vi "Do.vi"(8 "error in (no error)":errorcluster, 10 "Actor in":refnum<class "Actor.lvclass">, 11 "Launch Nested Panel Message Msg in":refnum<class "Launch Nested Panel Message Msg.lvclass">) -> (0 "error out":errorcluster, 2 "Actor out":refnum<class "Actor.lvclass">)   [LabVIEW 2023, in "Panel Actor.lvlib" / "Launch Nested Panel Message Msg.lvclass"]
doc: "(<B>Filename</B>: Actor Framework.lvlib:Message.lvclass:Do.vi)\n\nDefines what a message does when it is received by an actor. Generally, a message instructs an actor to invoke one of its methods. By default, this method does nothing. A child class must override it to define behavior. Create a child class by using the Actor Framework Message Maker dialog box."
uses:
  Launch Nested Panel Message Msg.lvclass
  builds/Framework/Actor Framework.lvlibp/1abvi3w/vi.lib/ActorFramework/Actor/Actor.lvclass
  Library/Panel Actor.lvclass
  C:/Users/Public/Documents/Development/builds/Framework/Actor Framework.lvlibp/1abvi3w/vi.lib/ActorFramework/Actor/Actor.lvclass
  Launch Nested Panel Message Msg.lvclass/Launch Nested Panel Message Msg.ctl
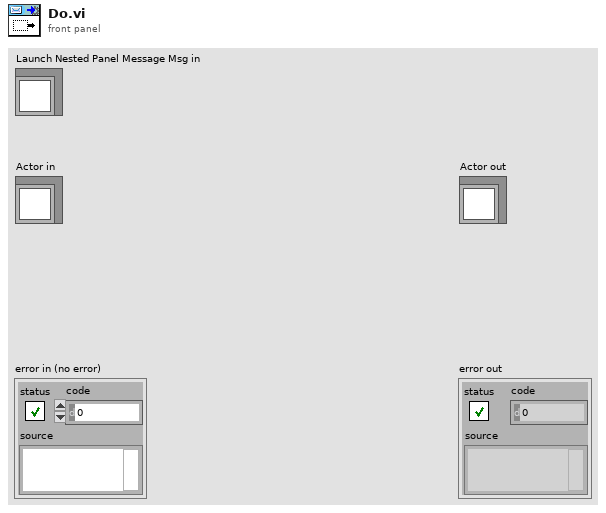
[diagram p1: front panel]
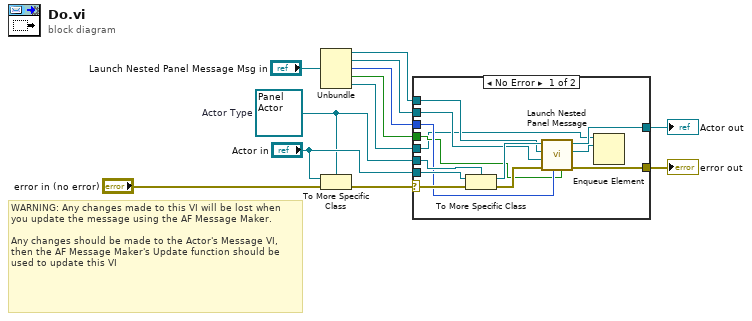
[diagram p0: block diagram]
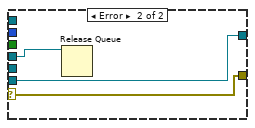
[diagram p2: hidden frame]
diagram:
  w7 = refnum<class "Panel Actor.lvclass"> refnum  # Actor Type
  # "WARNING: Any changes made to this VI will be lost when you update the message using the AF Message Maker.\n\nAny changes should be made to the Actor's Message VI, then the AF Message Maker's Update function should be used to update this VI"
  n1 = Unbundle("Launch Nested Panel Message Msg in") -> (w6:refnum<class "Panel Actor.lvclass">, w5:refnum<class "Panel.lvclass">, w4:i32, w3:bool, w1:refnum<queue>)
  n2 = To More Specific Class(target class=w7, reference="Actor in", error in="error in (no error)") -> (error out=w11:errorcluster)  [unwired: 1 out]
  n3 = case shown="No Error" w11 {
    selector: w11 -> [w25 w28]
    tunnel: [w20 w28] -> w10
    tunnel: [w19 w27] -> w9
    tunnel: "Actor in" -> [w24 w27]
    tunnel: w7 -> [w23 _]
    tunnel: w6 -> [w18 _]
    tunnel: w5 -> [w17 _]
    tunnel: w4 -> [w16 _]
    tunnel: w3 -> [w15 _]
    tunnel: w1 -> [w14 w26]
    frame No Error {
      n4 = To More Specific Class ("Actor Cast")(target class=w23, reference=w24, error in=w25) -> (specific class reference=w22:refnum<class "Panel Actor.lvclass">, error out=w21:errorcluster)
      n5 = call "Launch Nested Panel Message.vi"("Auto-stop? (T)"=w15, "timeout in ms (-1)"=w16, "error in (no error)"=w21, "Panel"=w17, "Nested Panel Actor"=w18, "Panel Actor in"=w22) -> ("error out"=w20:errorcluster, "Nested Actor's Enqueuer"=w13:refnum<class "Message Enqueuer.lvclass">, "Panel Actor out"=w19:refnum<class "Panel Actor.lvclass">)  [unwired: 3 in]
      n6 = Enqueue Element(queue=w14, element=w13) -> ()  [unwired: 2 in, 3 out]
    }
    frame Error {
      n7 = Release Queue(queue=w26) -> ()  [unwired: 2 in, 3 out]
    }
  }
  "error out" <- w10
  "Actor out" <- w9
